vi "Initialise.vi"(4 "Rate (Hz)":dbl=1000.0 format="%0.2f", 6 "WarmupIters":u32=2000, 8 "error in (no error)":errorcluster, 9 "Master Clock":tag, 10 "Tasks Info":T1[](array[typedef]), 11 "PXI in":refnum<class "PXI.lvclass">) -> (0 "error out":errorcluster, 3 "PXI out":refnum<class "PXI.lvclass">)   [LabVIEW 2011, in "PXI.lvclass"]
uses:
  PXI.lvclass
  controls/Task Definition.ctl
  controls/Task Types.ctl
  PXI.lvclass/PXI.ctl
  <vilib>/DAQmx/create/channels.llb/DAQmx Create Channel (AI-Voltage-Basic).vi
  <vilib>/DAQmx/configure/timing.llb/DAQmx Timing (Sample Clock).vi
  <vilib>/DAQmx/create/channels.llb/DAQmx Create Channel (AO-Voltage-Basic).vi
  <vilib>/DAQmx/create/channels.llb/DAQmx Create Channel (DI-Digital Input).vi
  <vilib>/DAQmx/create/channels.llb/DAQmx Create Channel (DO-Digital Output).vi
  Program Files/National Instruments/LabVIEW 2011/resource/objmgr/daqmx.rc
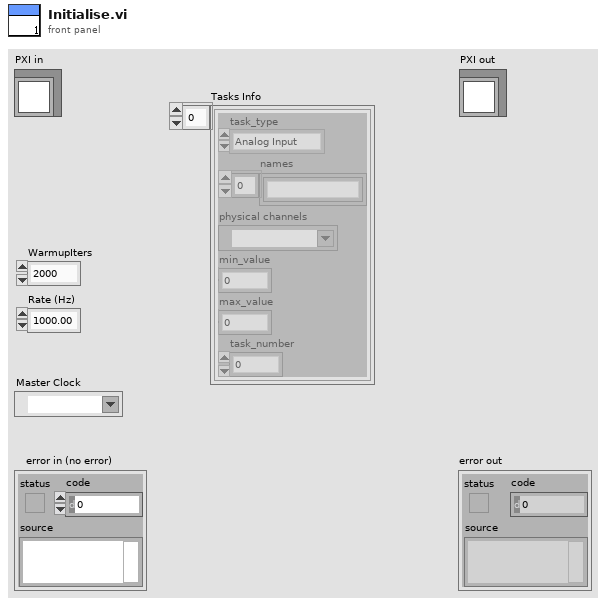
[diagram p1: front panel]
types:
  T1 = typedef "Task Definition.ctl" = cluster{"task_type":T2, "names":string[], "physical channels":tag, "min_value":dbl, "max_value":dbl, "task_number":i32}
  T2 = typedef "Task Types.ctl" = enum16{"Analog Input", "Analog Output", "Digital Input", "Digital Output"}
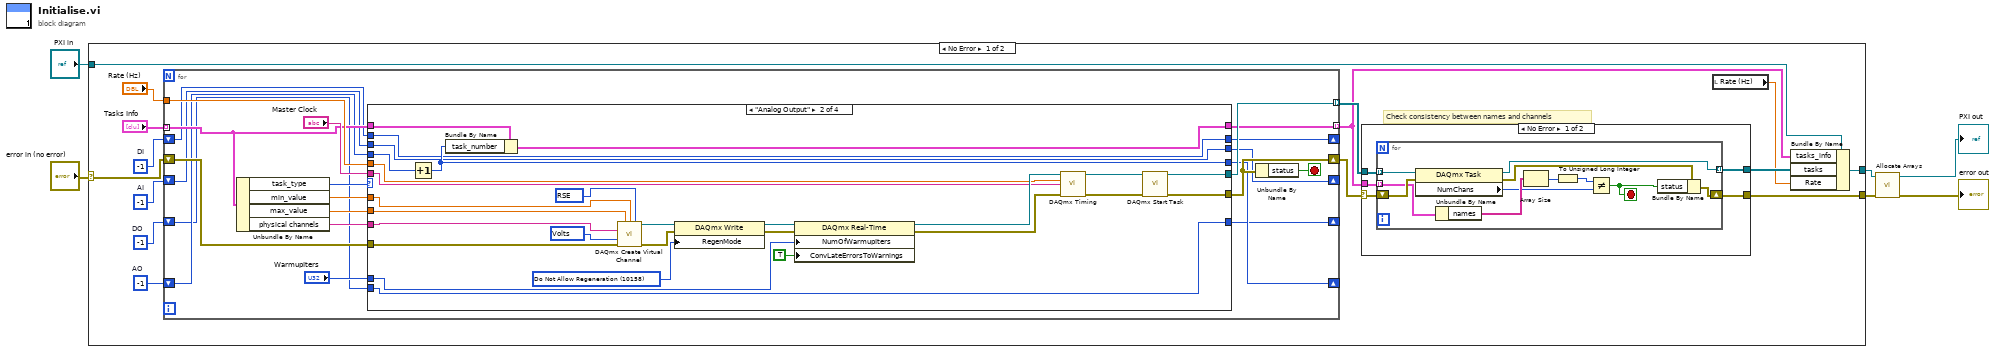
[diagram p0: block diagram]
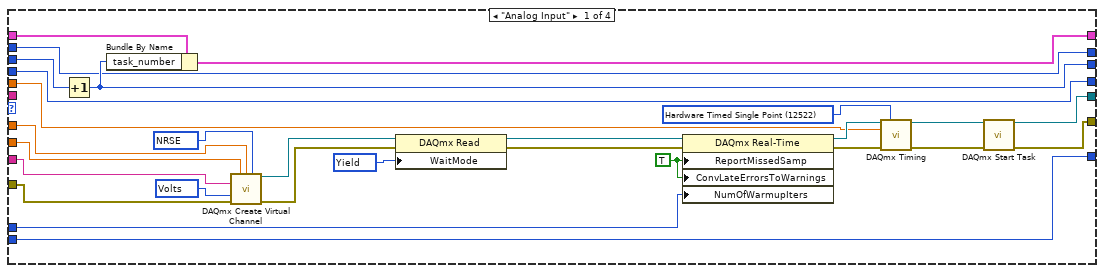
[diagram p3: hidden frame]
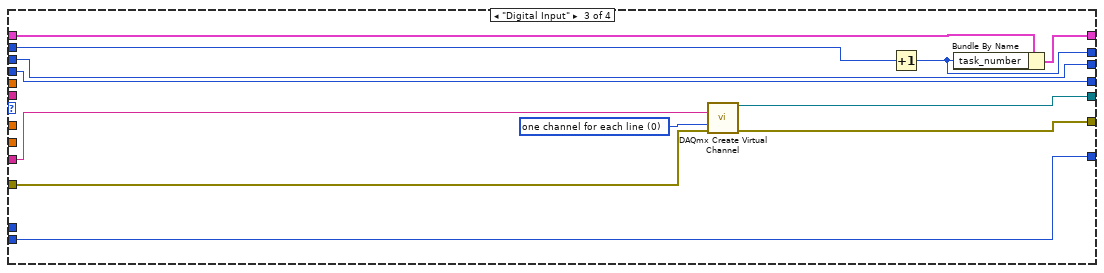
[diagram p4: hidden frame]
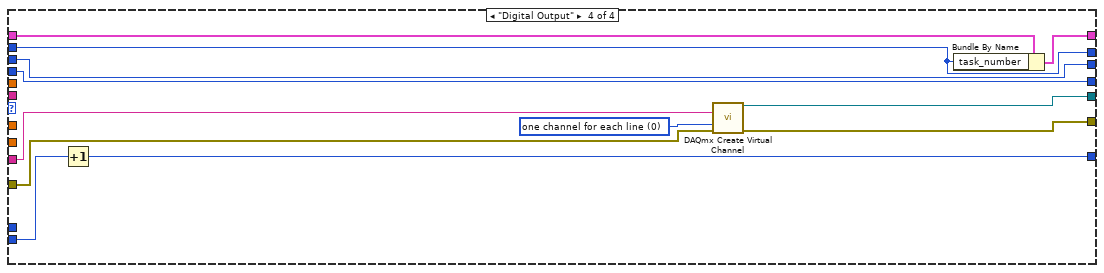
[diagram p5: hidden frame]
diagram:
  n1 = case shown="No Error" "error in (no error)" {
    selector: "error in (no error)" -> [w19 w142]
    tunnel: [w17 w142] -> w3
    tunnel: [w20 w141] -> w4
    tunnel: "PXI in" -> [w21 w141]
    frame No Error {
      w7 = -1  # DO
      w8 = -1  # DI
      w9 = -1  # AO
      w10 = -1  # AI
      # "Check consistency between names and channels"
      n2 = for {
        tunnel: "Tasks Info" -> [w48] mode=indexing
        tunnel: [w55] -> w16 mode=indexing
        shift-right: [w53] -> w18
        shift-left: w19 -> [w54]
        tunnel: "Rate (Hz)" -> [w50]
        tunnel: [w47] -> w11 mode=indexing
        shift-right: [w49] -> _
        shift-left: w10 -> [w46]
        shift-right: [w44] -> _
        shift-left: w9 -> [w45]
        shift-right: [w42] -> _
        shift-left: w8 -> [w43]
        shift-right: [w40] -> _
        shift-left: w7 -> [w41]
        stop <- w52 stop-if-true
        n3 = Unbundle By Name(w48) -> ("task_type"=w51:T2, "min_value"=w59:dbl, "max_value"=w58:dbl, "physical channels"=w57:tag)
        n4 = case shown="\"Analog Output\"" w51 {
          tunnel: w59 -> [w86 w103 _ _]
          tunnel: w58 -> [w85 w102 _ _]
          tunnel: w57 -> [w84 w96 w127 w139]
          tunnel: "WarmupIters" -> [w74 w106 _ _]
          tunnel: "Master Clock" -> [_ w105 _ _]
          tunnel: w50 -> [w73 w104 _ _]
          tunnel: [w70 w99 w126 w138] -> w55
          tunnel: [w69 w98 w125 w137] -> w53
          tunnel: w54 -> [w68 w97 w124 w136]
          tunnel: w46 -> [w67 w91 w123 w135]
          tunnel: [w65 w91 w123 w135] -> w49
          tunnel: w48 -> [w66 w94 w121 w132]
          tunnel: [w64 w93 w120 w133] -> w47
          tunnel: w45 -> [w63 w95 w122 w134]
          tunnel: [w63 w92 w122 w134] -> w44
          tunnel: w43 -> [w62 w90 w119 w129]
          tunnel: [w62 w90 w117 w129] -> w42
          tunnel: w41 -> [w61 w89 w118 w131]
          tunnel: [w61 w89 w118 w130] -> w40
          frame "Analog Input" {
            w75 = TRUE ("ConvLateErrorsToWarnings")
            w78 = 12522 items=["Finite Samples"=10178, "Continuous Samples"=10123, "Hardware Timed Single Point"=12522] ("sample mode")
            w83 = 12525 items=["Wait For Interrupt"=12523, "Poll"=12524, "Yield"=12525, "Sleep"=12547] ("WaitMode")
            w87 = 10348 items=["Volts"=10348, "From Custom Scale"=10065] ("units")
            w88 = 10078 items=["default"=-1, "RSE"=10083, "NRSE"=10078, "Differential"=10106, "Pseudodifferential"=12529] ("input terminal configuration")
            n5 = Increment(x=w67) -> (x+1=w65:i32)
            n6 = Bundle By Name(cluster=w66, "task_number"=w65) -> (w64:T1)
            n7 = call-poly <vilib>:"DAQmx Create Virtual Channel.vi"("maximum value"=w85, "minimum value"=w86, "input terminal configuration"=w88, "physical channels"=w84, "units"=w87, "error in"=w68) -> ("task out"=w77:refnum<k21>, "error out"=w76:errorcluster)  [unwired: 8 in]
            n8 = property class="DAQmx Read"(reference=w77, error in=w76, "WaitMode"=w83) -> (reference out=w81:refnum<k21>, error out=w82:errorcluster)
            n9 = property class="DAQmx Real-Time"(reference=w81, error in=w82, "ReportMissedSamp"=w75, "ConvLateErrorsToWarnings"=w75, "NumOfWarmupIters"=w74) -> (reference out=w79:refnum<k21>, error out=w80:errorcluster)
            n10 = call-poly <vilib>:"DAQmx Timing.vi"("task/channels in"=w79, "sample mode"=w78, "rate"=w73, "error in"=w80) -> ("task out"=w72:refnum<k21>, "error out"=w71:errorcluster)  [unwired: 10 in]
            n11 = call <vilib>:"DAQmx Start Task.vi"("task/channels in"=w72, "error in"=w71) -> ("task out"=w70:refnum<k21>, "error out"=w69:errorcluster)  [unwired: 12 in]
          }
          frame "Analog Output" {
            w113 = 10158 items=["Allow Regeneration"=10097, "Do Not Allow Regeneration"=10158] ("RegenMode")
            w116 = 10083 items=["Default"=-1, "RSE"=10083, "Differential"=10106, "Pseudodifferential"=12529] ("output terminal configuration")
            w115 = 10348 items=["Volts"=10348, "From Custom Scale"=10065] ("units")
            n12 = Increment(x=w95) -> (x+1=w92:i32)
            n13 = Bundle By Name(cluster=w94, "task_number"=w92) -> (w93:T1)
            n14 = call-poly <vilib>:"DAQmx Create Virtual Channel.vi"("maximum value"=w102, "minimum value"=w103, "output terminal configuration"=w116, "physical channels"=w96, "units"=w115, "error in"=w97) -> ("task out"=w112:refnum<k21>, "error out"=w111:errorcluster)  [unwired: 8 in]
            n15 = property class="DAQmx Write"(reference=w112, error in=w111, "RegenMode"=w113) -> (reference out=w110:refnum<k21>, error out=w109:errorcluster)
            n16 = property class="DAQmx Real-Time"(reference=w110, error in=w109, "NumOfWarmupIters"=w106, "ConvLateErrorsToWarnings"=TRUE ("ReportMissedSamp")) -> (reference out=w108:refnum<k21>, error out=w107:errorcluster)
            n17 = call-poly <vilib>:"DAQmx Timing.vi"("task/channels in"=w108, "rate"=w104, "source"=w105, "error in"=w107) -> ("task out"=w101:refnum<k21>, "error out"=w100:errorcluster)  [unwired: 10 in]
            n18 = call <vilib>:"DAQmx Start Task.vi"("task/channels in"=w101, "error in"=w100) -> ("task out"=w99:refnum<k21>, "error out"=w98:errorcluster)  [unwired: 12 in]
          }
          frame "Digital Input" {
            w128 = 0 items=["one channel for each line", "one channel for all lines"] ("line grouping")
            n19 = call-poly <vilib>:"DAQmx Create Virtual Channel.vi"("lines"=w127, "line grouping"=w128, "error in"=w124) -> ("task out"=w126:refnum<k21>, "error out"=w125:errorcluster)  [unwired: 11 in]
            n20 = Increment(x=w119) -> (x+1=w117:i32)
            n21 = Bundle By Name(cluster=w121, "task_number"=w117) -> (w120:T1)
          }
          frame "Digital Output" {
            w140 = 0 items=["one channel for each line", "one channel for all lines"] ("line grouping")
            n22 = Increment(x=w131) -> (x+1=w130:i32)
            n23 = call-poly <vilib>:"DAQmx Create Virtual Channel.vi"("lines"=w139, "line grouping"=w140, "error in"=w136) -> ("task out"=w138:refnum<k21>, "error out"=w137:errorcluster)  [unwired: 11 in]
            n24 = Bundle By Name(cluster=w132, "task_number"=w129) -> (w133:T1)
          }
        }
        n25 = Unbundle By Name(w53) -> ("status"=w52:bool)
      }
      n26 = case shown="No Error" w18 {
        selector: w18 -> [w24 w39]
        tunnel: [w22 w39] -> w17
        tunnel: w16 -> [w25 w38]
        tunnel: w11 -> [w26 _]
        tunnel: [w23 w38] -> w14
        frame No Error {
          n27 = for {
            tunnel: w26 -> [w35] mode=indexing
            tunnel: w25 -> [w37] mode=indexing
            tunnel: [w30] -> w23 mode=indexing
            shift-right: [w28] -> w22
            shift-left: w24 -> [w36]
            stop <- w27 stop-if-true
            n28 = property class="DAQmx Task"(reference=w37, error in=w36) -> (reference out=w30:refnum<k21>, error out=w29:errorcluster, "NumChans"=w33:u32)
            n29 = Unbundle By Name(w35) -> ("names"=w34:string[])
            n30 = Array Size(array=w34) -> (size(s)=w32:i32)
            n31 = To Unsigned Long Integer(number=w32) -> (unsigned 32bit integer=w31:u32)
            n32 = Not Equal?(x=w31, y=w33) -> (x != y?=w27:bool)
            n33 = Bundle By Name(cluster=w29, "status"=w27) -> (w28:errorcluster)
          }
        }
        frame Error {
        }
      }
      n34 = local read "Rate (Hz)"() -> (w12:dbl)
      n35 = Bundle By Name(cluster=w21, "tasks_info"=w11, "tasks"=w14, "Rate"=w12) -> (w20:refnum<class "PXI.lvclass">)
    }
    frame Error {
    }
  }
  n36 = call "Allocate Arrays.vi"("error in (no error)"=w3, "PXI in"=w4) -> ("error out"=→"error out":errorcluster, "PXI out"=→"PXI out":refnum<class "PXI.lvclass">)  [unwired: 8 in]
